vi "Auto Vision V.5.0.vi"() -> ()   [LabVIEW 2016]
uses:
  <vilib>/Rock Robotics/WPI/Utilities/WPI_GetSetVariantRefNum.vi
  Robot Global Data V.5.0.vi
panel:
  out "Ideal Center":dbl
  in  "Right Speed Fix":dbl format="%#_13g"
  in  "Left Speed Fix":dbl format="%#_13g"
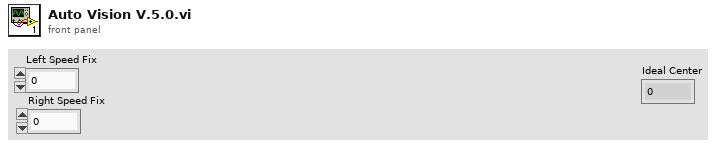
[diagram p1: front panel]
types:
  T1 = cluster{"Distance (ft)":dbl, "Score":dbl, "Normalized":cluster{"Center":cluster{dbl, dbl}, "Rectangle":cluster{"Numeric":dbl, "Numeric 2":dbl, "Numeric 3":dbl, "Numeric 5":dbl}}, "Pixels":cluster{"Center":cluster{dbl, dbl}, "Rectangle":cluster{"Numeric":dbl, "Numeric 2":dbl, "Numeric 3":dbl, "Numeric 5":dbl}}}
  T2 = cluster{"Center":cluster{dbl, dbl}, "Rectangle":cluster{"Numeric":dbl, "Numeric 2":dbl, "Numeric 3":dbl, "Numeric 5":dbl}}
  T3 = typedef "WPI_RobotDriveDevRef.ctl" = cluster{"DevStatus":errorcluster, "Motors[]":T4[], "Square Inputs":bool, "Max Output":dbl}
  T4 = typedef "WPI_MotorControlDeviceRef.ctl" = cluster{"DeviceStatus":errorcluster, "Type":T5, "PWM":cluster{"PWM Channel":T6, "DeadBand":T7}, "CAN":cluster{"Device Number":u8, "SetOutput VI Ref":variant, "GetOutput VI Ref":variant, "Enable VI Ref":variant, "Disable VI Ref":variant, "Data":variant}, "Invert":bool}
  T5 = typedef "WPI_MotorControlType.ctl" = enum16{"PWM", "CAN"}
  T6 = typedef "FPGA_DIOPWMChannel.ctl" = enum8{"PWM 0", "PWM 1", "PWM 2", "PWM 3", "PWM 4", "PWM 5", "PWM 6", "PWM 7", "PWM 8", "PWM 9", "PWM MXP 0", "PWM MXP 1", "PWM MXP 2", "PWM MXP 3", "PWM MXP 4", "PWM MXP 5", "PWM MXP 6", "PWM MXP 7", "PWM MXP 8", "PWM MXP 9", "Invalid"}
  T7 = typedef "WPI_PWMDeadband.ctl" = cluster{"Name":string, "maxPositivePwm":i32, "minPositivePwm":i32, "centerPwm":i32, "maxNegativePwm":i32, "minNegativePwm":i32, "angularRange":u16}
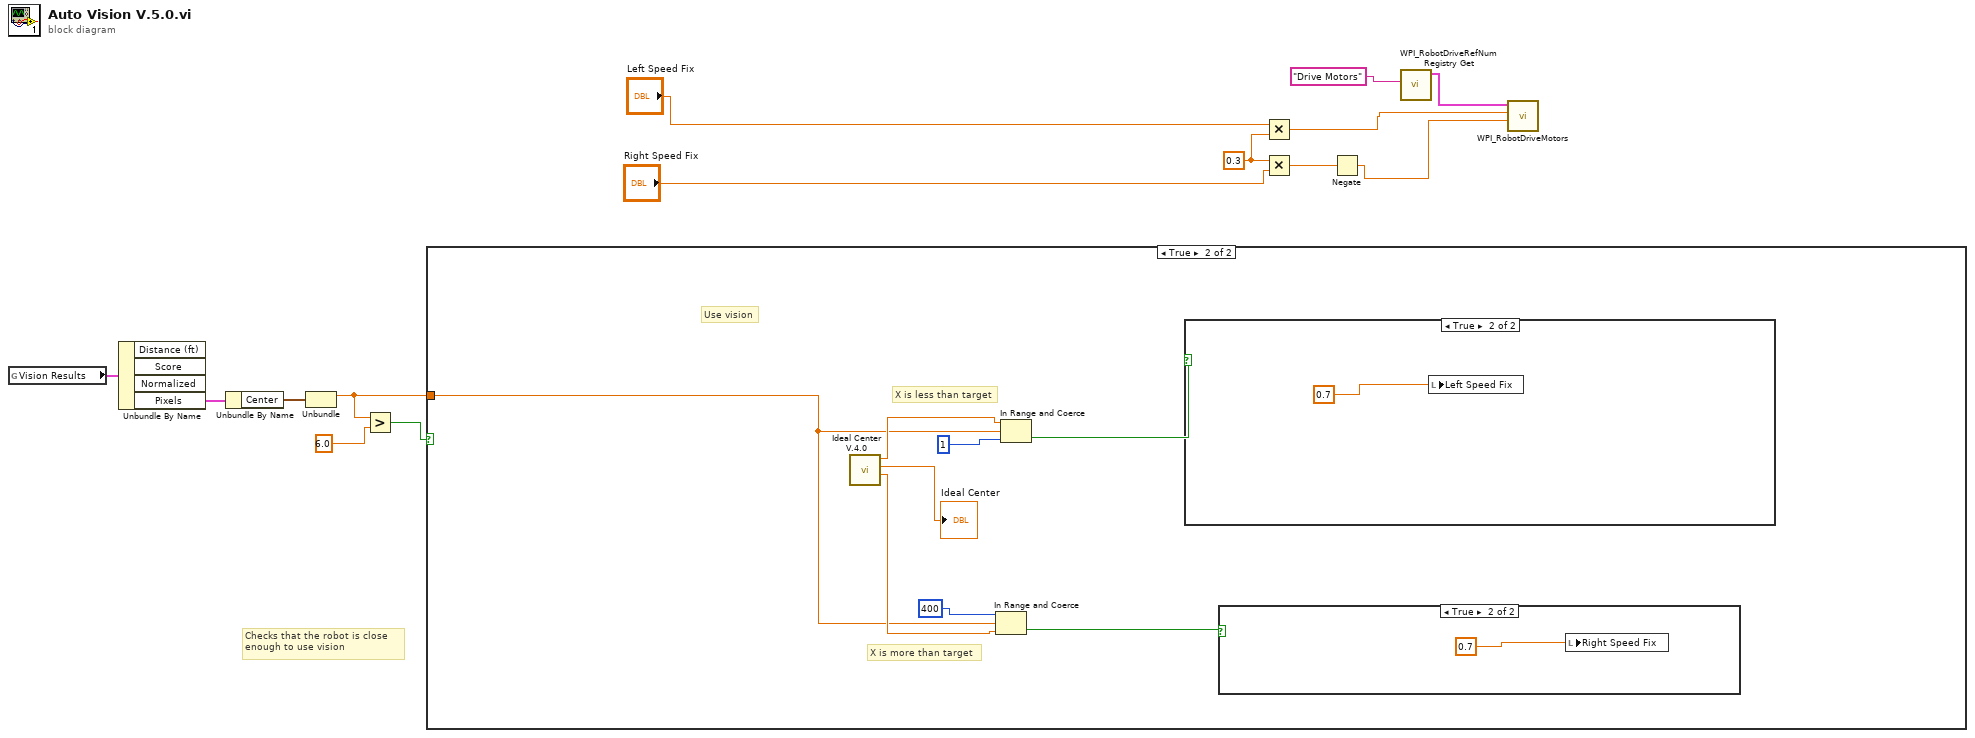
[diagram p0: block diagram]
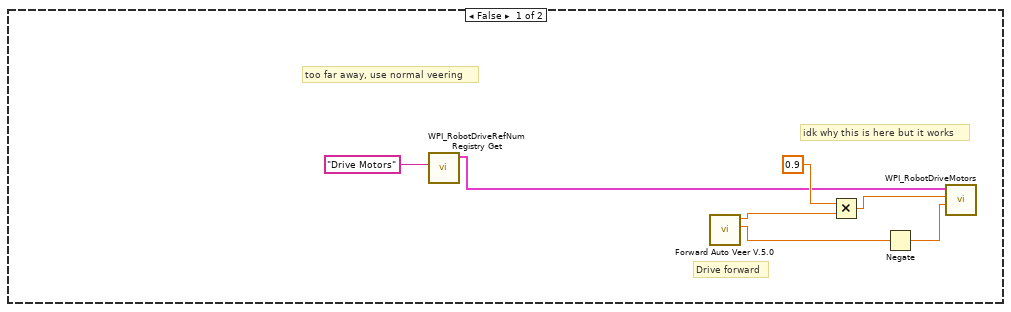
[diagram p2: hidden frame]
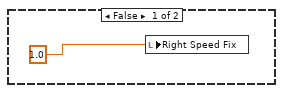
[diagram p3: hidden frame]
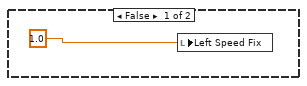
[diagram p4: hidden frame]
diagram:
  w14 = 0.3
  # "Checks that the robot is close \nenough to use vision"
  n1 = global read "Robot Global Data V.5.0.vi" "Vision Results"() -> (w8:T1)
  n2 = Unbundle By Name(w8) -> ("Pixels"=w9:T2)  [unwired: 3 out]
  n3 = Unbundle By Name(w9) -> ("Center"=w10:cluster{dbl, dbl})
  n4 = Unbundle(w10) -> (w6:dbl)  [unwired: 1 out]
  n5 = Greater?(x=w6, y=6.0) -> (0:w7:bool)
  n6 = case shown="True" w7 {
    tunnel: w6 -> [_ w23]
    frame False {
      # "idk why this is here but it works"
      # "Drive forward"
      # "too far away, use normal veering"
      n7 = call <vilib>:"WPI_RobotDriveRefNum Registry Get.vi"("refnum name"="Drive Motors") -> ("RobotDriveDevRef"=w15:T3)  [unwired: 9 in, 1 out]
      n8 = call "Forward Auto Veer V.5.0.vi"() -> ("Right"=w20:dbl, "Left"=w19:dbl)  [unwired: 10 in]
      n9 = Multiply(x=0.9, y=w19) -> (x*y=w17:dbl)
      n10 = Negate(x=w20) -> (-x=w21:dbl)
      n11 = call <vilib>:"WPI_RobotDriveMotors.vi"("RightSpeed"=w21, "LeftSpeed"=w17, "RobotDriveDevRef"=w15) -> ()  [unwired: 6 in, 3 out]
    }
    frame True {
      # "Use vision"
      # "X is less than target"
      # "X is more than target"
      n12 = call "Ideal Center V.4.0.vi"() -> ("Center+1"=w24:dbl, "Ideal Center"=→"Ideal Center":dbl, "Center-1"=w25:dbl)  [unwired: 9 in]
      n13 = In Range and Coerce(upper limit=400, x=w23, lower limit=w24) -> (In Range?=w26:bool)  [unwired: 1 out]
      n14 = In Range and Coerce(upper limit=w25, x=w23, lower limit=1) -> (In Range?=w29:bool)  [unwired: 1 out]
      n15 = case shown="True" w29 {
        frame False {
          n16 = local write "Left Speed Fix"(1.0) -> ()
        }
        frame True {
          n17 = local write "Left Speed Fix"(0.7) -> ()
        }
      }
      n18 = case shown="True" w26 {
        frame False {
          n19 = local write "Right Speed Fix"(1.0) -> ()
        }
        frame True {
          n20 = local write "Right Speed Fix"(0.7) -> ()
        }
      }
    }
  }
  n21 = Multiply(x="Left Speed Fix", y=w14) -> (x*y=w3:dbl)
  n22 = Multiply(x=w14, y="Right Speed Fix") -> (x*y=w13:dbl)
  n23 = Negate(x=w13) -> (-x=w2:dbl)
  n24 = call <vilib>:"WPI_RobotDriveRefNum Registry Get.vi"("refnum name"="Drive Motors") -> ("RobotDriveDevRef"=w1:T3)  [unwired: 9 in, 1 out]
  n25 = call <vilib>:"WPI_RobotDriveMotors.vi"("RightSpeed"=w2, "LeftSpeed"=w3, "RobotDriveDevRef"=w1) -> ()  [unwired: 6 in, 3 out]
